vi "Query System Status.vi"(6 "timeout (ms)":i32=5000, 7 "Plugin Name":string, 8 "error in":errorcluster, 9 "channels.channels":T1[](array[typedef]), 10 "Status":T6 {"Monitor Doubles"."4" format="%#_9g"; "Monitor Doubles"."3" format="%#_9g"; "Monitor Doubles"."2" format="%#_9g"; "Monitor Doubles"."1" format="%#_9g"}, 11 "gRPC ID in":T15) -> (0 "error out":errorcluster, 2 "Clock Conversion Array":T4[](array[typedef]), 3 "gRPC ID out":T15)   [LabVIEW 2021, in "CIFManagerClientWrapper.lvlib"]
uses:
  CIFManagerClientWrapper.lvlib
  <vilib>/gRPC/LabVIEW gRPC Library/Shared/grpcId.ctl
  CIFCore/Common/Typedef/Plugin Status.ctl
  CIFCore/Common/Typedef/Plugin State.ctl
  CIFCore/Common/Typedef/Timing Statistics.ctl
  CIFCore/Common/Typedef/Timing Stats Base.ctl
  CIFCore/Common/Typedef/FIFO Statistics.ctl
  CIFCore/Common/Typedef/Simple Error.ctl
  CIFCore/Common/Typedef/Monitor Doubles.ctl
  CIFCore/Common/Typedef/Monitor U64.ctl
  CIFCore/Common/Typedef/Monitor I64.ctl
  <vilib>/CIF Foundation/CIF Utilities/Time/Typedef/Clock Conversion.ctl
  <vilib>/CIF Foundation/CIF Utilities/Time/Typedef/Timestamp Pair.ctl
  CIF_Manager_client/RPC Messages/cif_management_common_Channel.ctl
  CIF_Manager_client/RPC Messages/cif_management_common_ChannelDirection.ctl
  CIF_Manager_client/RPC Messages/cif_management_common_ChannelPattern.ctl
  CIF_Manager_client/RPC Messages/cif_manager_QuerySystemStatusRequest.ctl
  CIF_Manager_client/RPC Messages/cif_manager_PluginStatus.ctl
  CIF_Manager_client/RPC Messages/cif_management_common_PluginStatusData.ctl
  CIF_Manager_client/RPC Messages/cif_management_common_PluginStatusData_PluginState.ctl
  CIF_Manager_client/RPC Messages/cif_management_common_TimingStatistics.ctl
  CIF_Manager_client/RPC Messages/cif_common_TimingStats.ctl
  CIF_Manager_client/RPC Messages/cif_management_common_FifoStatistics.ctl
  CIF_Manager_client/RPC Messages/cif_management_common_Error.ctl
  CIF_Manager_client/RPC Messages/cif_management_common_MonitorDoubles.ctl
  CIF_Manager_client/RPC Messages/cif_management_common_MonitorU64.ctl
  CIF_Manager_client/RPC Messages/cif_management_common_MonitorI64.ctl
  CIF_Manager_client/RPC Messages/cif_management_common_Channels.ctl
  CIF_Manager_client/CIF_Manager_client.lvlib
  <vilib>/CIF Foundation/CIF Utilities/Time/Time_CIF_U.lvlib
  CIFCore/Grpc/CIFCoreWrapper/CIFCoreWrapper.lvlib
  <vilib>/gRPC/LabVIEW gRPC Library/grpc-lvsupport-release.lvlib
  CIFCore/Common/CIFCoreCommon.lvlib
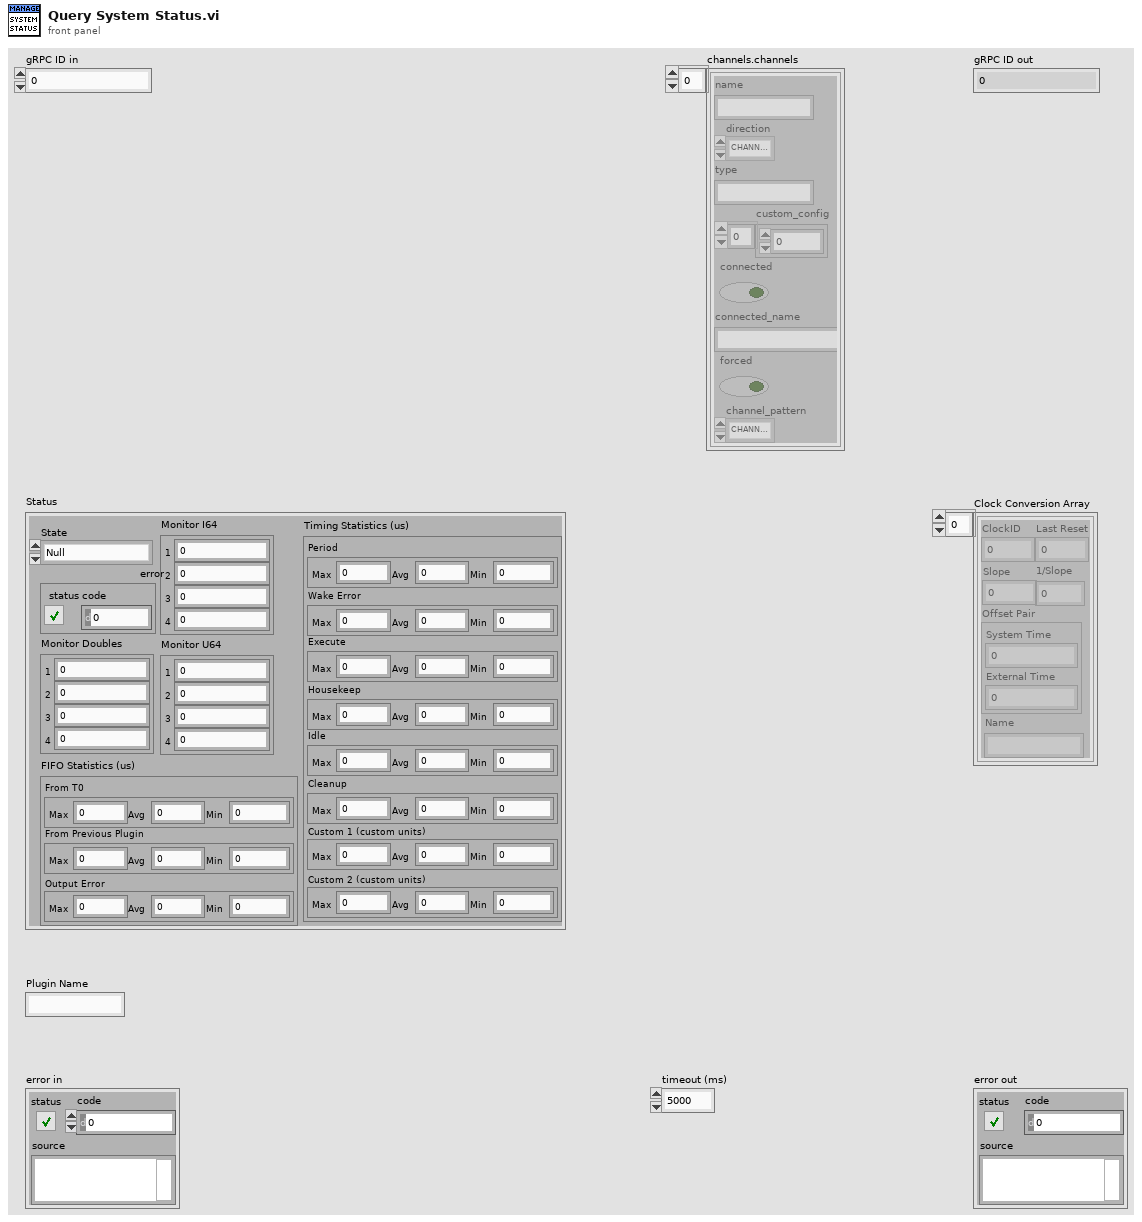
[diagram p1: front panel]
types:
  T1 = typedef "CIF_Manager_client.lvlib/cif_management_common_Channel.ctl" = cluster{"name":string, "direction":T2, "type":string, "custom_config":u8[], "connected":bool, "connected_name":string, "forced":bool, "channel_pattern":T3}
  T2 = typedef "CIF_Manager_client.lvlib/cif_management_common_ChannelDirection.ctl" = enum32{"CHANNELDIRECTION_UNKNOWN", "CHANNELDIRECTION_PUBLISHER", "CHANNELDIRECTION_SUBSCRIBER"}
  T3 = typedef "CIF_Manager_client.lvlib/cif_management_common_ChannelPattern.ctl" = enum32{"CHANNELPATTERN_UNKNOWN", "CHANNELPATTERN_TAG", "CHANNELPATTERN_FIFO", "CHANNELPATTERN_MULTIFIFO", "CHANNELPATTERN_BACKPRESSUREFIFO"}
  T4 = typedef "Time_CIF_U.lvlib/Clock Conversion.ctl" = cluster{"ClockID":u8, "Last Reset":i64, "Offset Pair":T5, "Slope":dbl, "1/Slope":dbl, "Name":string}
  T5 = typedef "Time_CIF_U.lvlib/Timestamp Pair.ctl" = cluster{"System Time":i64, "External Time":i64}
  T6 = typedef "CIFCoreCommon.lvlib/Plugin Status.ctl" = cluster{"State":T7, "Timing Statistics (us)":T8, "FIFO Statistics (us)":T10, "error":T11, "Monitor Doubles":T12, "Monitor U64":T13, "Monitor I64":T14}
  T7 = typedef "CIFCoreCommon.lvlib/Plugin State.ctl" = enum32{"Null", "Creating", "Listening", "Running", "CleaningUp", "Destroying"}
  T8 = typedef "CIFCoreCommon.lvlib/Timing Statistics.ctl" = cluster{"Period":T9, "Wake Error":T9, "Execute":T9, "Housekeep":T9, "Idle":T9, "Cleanup":T9, "Custom 1 (custom units)":T9, "Custom 2 (custom units)":T9}
  T9 = typedef "CIFCoreCommon.lvlib/Timing Stats Base.ctl" = cluster{"Max":i64, "Avg":dbl, "Min":i64}
  T10 = typedef "CIFCoreCommon.lvlib/FIFO Statistics.ctl" = cluster{"From T0":T9, "From Previous Plugin":T9, "Output Error":T9}
  T11 = typedef "CIFCoreCommon.lvlib/Simple Error.ctl" = cluster{"status":bool, "code":i32}
  T12 = typedef "CIFCoreCommon.lvlib/Monitor Doubles.ctl" = cluster{"1":dbl, "2":dbl, "3":dbl, "4":dbl}
  T13 = typedef "CIFCoreCommon.lvlib/Monitor U64.ctl" = cluster{"1":u64, "2":u64, "3":u64, "4":u64}
  T14 = typedef "CIFCoreCommon.lvlib/Monitor I64.ctl" = cluster{"1":i64, "2":i64, "3":i64, "4":i64}
  T15 = typedef "grpc-lvsupport-release.lvlib/grpcId.ctl" = u64
  T16 = typedef "CIF_Manager_client.lvlib/cif_manager_QuerySystemStatusRequest.ctl" = cluster{"plugin_status":T17}
  T17 = typedef "CIF_Manager_client.lvlib/cif_manager_PluginStatus.ctl" = cluster{"pluginname":string, "status":T18, "channels":T27}
  T18 = typedef "CIF_Manager_client.lvlib/cif_management_common_PluginStatusData.ctl" = cluster{"state":T19, "timing_statistics":T20, "fifo_statistics":T22, "error":T23, "monitor_doubles":T24, "monitor_u64s":T25, "monitor_i64s":T26}
  T19 = typedef "CIF_Manager_client.lvlib/cif_management_common_PluginStatusData_PluginState.ctl" = enum32{"PLUGINSTATE_UNKNOWN", "PLUGINSTATE_CREATING", "PLUGINSTATE_LISTENING", "PLUGINSTATE_RUNNING", "PLUGINSTATE_CLEANINGUP", "PLUGINSTATE_DESTROYING"}
  T20 = typedef "CIF_Manager_client.lvlib/cif_management_common_TimingStatistics.ctl" = cluster{"period":T21, "wake_error":T21, "execute":T21, "housekeep":T21, "idle":T21, "cleanup":T21, "custom_1":T21, "custom_2":T21}
  T21 = typedef "CIF_Manager_client.lvlib/cif_common_TimingStats.ctl" = cluster{"max":i64, "min":i64, "avg":dbl}
  T22 = typedef "CIF_Manager_client.lvlib/cif_management_common_FifoStatistics.ctl" = cluster{"from_t0":T21, "from_previous_plugin":T21, "output_error":T21}
  T23 = typedef "CIF_Manager_client.lvlib/cif_management_common_Error.ctl" = cluster{"status":bool, "code":i32}
  T24 = typedef "CIF_Manager_client.lvlib/cif_management_common_MonitorDoubles.ctl" = cluster{"double_1":dbl, "double_2":dbl, "double_3":dbl, "double_4":dbl}
  T25 = typedef "CIF_Manager_client.lvlib/cif_management_common_MonitorU64.ctl" = cluster{"u64_1":u64, "u64_2":u64, "u64_3":u64, "u64_4":u64}
  T26 = typedef "CIF_Manager_client.lvlib/cif_management_common_MonitorI64.ctl" = cluster{"i64_1":i64, "i64_2":i64, "i64_3":i64, "i64_4":i64}
  T27 = typedef "CIF_Manager_client.lvlib/cif_management_common_Channels.ctl" = cluster{"channels":T1[]}
  T28 = typedef "CIFCorePlugin_client.lvlib/cif_management_common_PluginStatusData.ctl" = cluster{"state":T29, "timing_statistics":T30, "fifo_statistics":T32, "error":T33, "monitor_doubles":T34, "monitor_u64s":T35, "monitor_i64s":T36}
  T29 = typedef "CIFCorePlugin_client.lvlib/cif_management_common_PluginStatusData_PluginState.ctl" = enum32{"PLUGINSTATE_UNKNOWN", "PLUGINSTATE_CREATING", "PLUGINSTATE_LISTENING", "PLUGINSTATE_RUNNING", "PLUGINSTATE_CLEANINGUP", "PLUGINSTATE_DESTROYING"}
  T30 = typedef "CIFCorePlugin_client.lvlib/cif_management_common_TimingStatistics.ctl" = cluster{"period":T31, "wake_error":T31, "execute":T31, "housekeep":T31, "idle":T31, "cleanup":T31, "custom_1":T31, "custom_2":T31}
  T31 = typedef "CIFCorePlugin_client.lvlib/cif_common_TimingStats.ctl" = cluster{"max":i64, "min":i64, "avg":dbl}
  T32 = typedef "CIFCorePlugin_client.lvlib/cif_management_common_FifoStatistics.ctl" = cluster{"from_t0":T31, "from_previous_plugin":T31, "output_error":T31}
  T33 = typedef "CIFCorePlugin_client.lvlib/cif_management_common_Error.ctl" = cluster{"status":bool, "code":i32}
  T34 = typedef "CIFCorePlugin_client.lvlib/cif_management_common_MonitorDoubles.ctl" = cluster{"double_1":dbl, "double_2":dbl, "double_3":dbl, "double_4":dbl}
  T35 = typedef "CIFCorePlugin_client.lvlib/cif_management_common_MonitorU64.ctl" = cluster{"u64_1":u64, "u64_2":u64, "u64_3":u64, "u64_4":u64}
  T36 = typedef "CIFCorePlugin_client.lvlib/cif_management_common_MonitorI64.ctl" = cluster{"i64_1":i64, "i64_2":i64, "i64_3":i64, "i64_4":i64}
  T37 = typedef "CIF_Manager_client.lvlib/cif_manager_QuerySystemStatusResponse.ctl" = cluster{"system_status":T38}
  T38 = typedef "CIF_Manager_client.lvlib/cif_manager_SystemStatus.ctl" = cluster{"clock_conversion_array":T39}
  T39 = typedef "CIF_Manager_client.lvlib/cif_manager_ClockConversionArray.ctl" = cluster{"clock_conversions":T40[]}
  T40 = typedef "CIF_Manager_client.lvlib/cif_manager_ClockConversion.ctl" = cluster{"clock_id":u32, "last_reset":i64, "slope":dbl, "offset_pair":T41, "clock_name":string}
  T41 = typedef "CIF_Manager_client.lvlib/cif_manager_TimePair.ctl" = cluster{"system_time":i64, "external_time":i64}
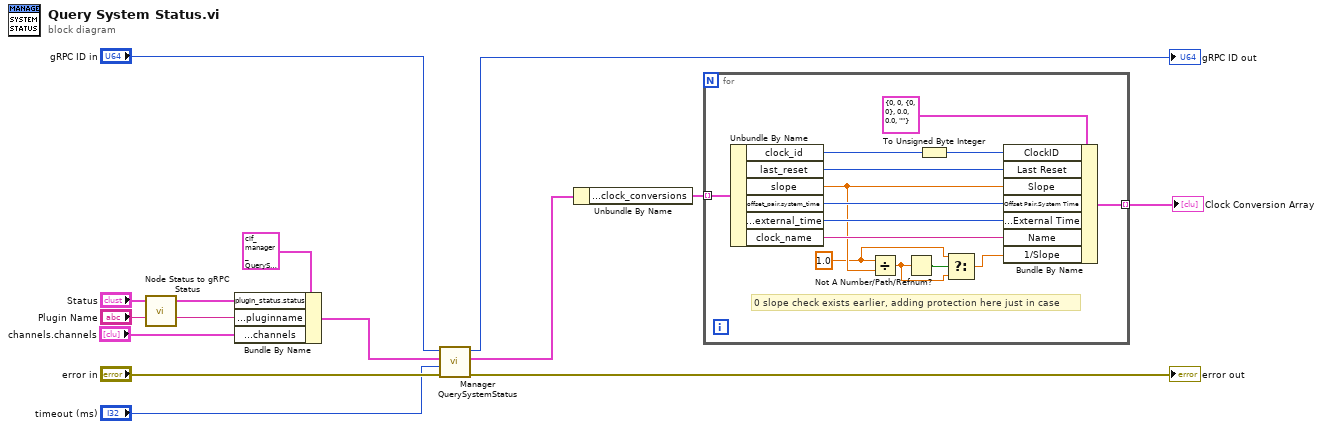
[diagram p0: block diagram]
diagram:
  n1 = call "Node Status to gRPC Status.vi"("Node Status"="Status") -> ("gRPC Status"=w5:T28)  [unwired: 3 in]
  n2 = Bundle By Name(cluster=T16 {"plugin_status"={"pluginname"="", "status"={"state"=enum."PLUGINSTATE_UNKNOWN", "timing_statistics"={"period"={"max"=0, "min"=0, "avg"=0.0}, "wake_error"={"max"=0, "min"=0, "avg"=0.0}, "execute"={"max"=0, "min"=0, "avg"=0.0}, "housekeep"={"max"=0, "min"=0, "avg"=0.0}, "idle"={"max"=0, "min"=0, "avg"=0.0}, "cleanup"={"max"=0, "min"=0, "avg"=0.0}, "custom_1"={"max"=0, "min"=0, "avg"=0.0}, "custom_2"={"max"=0, "min"=0, "avg"=0.0}}, "fifo_statistics"={"from_t0"={"max"=0, "min"=0, "avg"=0.0}, "from_previous_plugin"={"max"=0, "min"=0, "avg"=0.0}, "output_error"={"max"=0, "min"=0, "avg"=0.0}}, "error"={"status"=FALSE, "code"=0}, "monitor_doubles"={"double_1"=0.0, "double_2"=0.0, "double_3"=0.0, "double_4"=0.0}, "monitor_u64s"={"u64_1"=0, "u64_2"=0, "u64_3"=0, "u64_4"=0}, "monitor_i64s"={"i64_1"=0, "i64_2"=0, "i64_3"=0, "i64_4"=0}}, "channels"={"channels"=[]}}} ("Request Data"), "plugin_status.status"=w5, "plugin_status.pluginname"="Plugin Name", "plugin_status.channels.channels"="channels.channels") -> (w1:T16)
  n3 = call "Manager QuerySystemStatus.vi"("error in"="error in", "timeout (ms)"="timeout (ms)", "Request Data"=w1, "gRPC ID"="gRPC ID in") -> ("error out"=→"error out":errorcluster, "Response Data"=w8:T37, "gRPC ID out"=→"gRPC ID out":T15)  [unwired: 5 in]
  n4 = Unbundle By Name(w8) -> ("system_status.clock_conversion_array.clock_conversions"=w7:T40[])
  n5 = for {
    tunnel: w7 -> [w28] mode=indexing
    tunnel: [w21] -> w6 mode=indexing
    w16 = 1.0 ("x")
    # "0 slope check exists earlier, adding protection here just in case"
    n6 = Unbundle By Name(w28) -> ("clock_id"=w27:u32, "last_reset"=w24:i64, "slope"=w19:dbl, "offset_pair.system_time"=w23:i64, "offset_pair.external_time"=w22:i64, "clock_name"=w25:string)
    n7 = Divide(x=w16, y=w19) -> (x/y=w17:dbl)
    n8 = Not A Number/Path/Refnum?(number/path/refnum=w17) -> (NaN/Path/Refnum?=w18:bool)
    n9 = To Unsigned Byte Integer(number=w27) -> (unsigned 8bit integer=w26:u8)
    n10 = Select(t=w16, s=w18, f=w17) -> (s? t:f=w15:dbl)
    n11 = Bundle By Name(cluster=T4 {"ClockID"=0, "Last Reset"=0, "Offset Pair"={"System Time"=0, "External Time"=0}, "Slope"=0.0, "1/Slope"=0.0, "Name"=""} ("Clock Conversion"), "ClockID"=w26, "Last Reset"=w24, "Slope"=w19, "Offset Pair.System Time"=w23, "Offset Pair.External Time"=w22, "Name"=w25, "1/Slope"=w15) -> (w21:T4)
  }
  "Clock Conversion Array" <- w6
